vi "Clock Cross Retrieve.vi"(2 "resources":T2) -> (4 "read completion out":T1)   [LabVIEW 2020]
doc: "Retrieves the read completion from the other clock domain.\n\n<B>Input Parameters</B>\n\n<B>resources</B> contains references to the clock crossing FIFOs.\n\n<B>reset</B> is the register bus's reset signal.\n\n<B>Output Parameters</B>\n\n<B>read completion</B> the read completion data from the other clock domain.\n\n<B>ready for input</B> is a flow control signal that indicates whether the other clock domain's process is ready to accept a new instruction."
uses:
  Clock Cross Resources.ctl
  <instrlib>/_niInstr/Register Bus/v1/FPGA/Public/Read Completion.ctl
  <vilib>/rvi/DataTransferAndStorage/Container/Common/niFpgaContainerExecOnDevCompGetState.vi
  <vilib>/rvi/Emulation/niFpgaEmulationIsFPGAContextNoSignature.vi
  <vilib>/rvi/DataTransferAndStorage/Container/Common/niFpgaContainerGetUniqueNameForEmu.vi
  <vilib>/rvi/eio/common/nirviEmuReportErrorAndStop.vi
  <vilib>/rvi/Emulation/niFpgaSctlEmulationGetInTimedLoop.vi
  <vilib>/rvi/Emulation/niFpgaProcessEmulError.vi
  <vilib>/rvi/DataTransferAndStorage/Container/XNode/niFpgaContainer.xnode
  <vilib>/rvi/DataTransferAndStorage/Handshake/Emulation/niFpgaHandshakeEmulationRefIn.vi
  <instrlib>/_niInstr/Register Bus/v1/FPGA/niInstr Register Bus v1 FPGA.lvlib
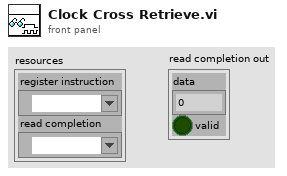
[diagram p1: front panel]
types:
  T1 = typedef "niInstr Register Bus v1 FPGA.lvlib/Read Completion.ctl" = cluster{"data":u32, "valid":bool}
  T2 = typedef "Clock Cross Resources.ctl" = cluster{"register instruction":refnum<k21>, "read completion":refnum<k21>}
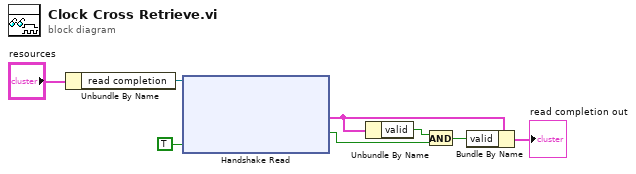
[diagram p0: block diagram]
diagram:
  n1 = Unbundle By Name("resources") -> ("read completion"=w4:refnum<k21>)
  n2 = xnode "Handshake Read"("Ready for Output"=TRUE ("ready for output"), "Handshake In"=w4) -> ("Data"=w1:cluster{"data":u32, "valid":bool}, "Output Valid"=w2:bool)  [unwired: 1 out]
  n3 = Unbundle By Name(w1) -> ("valid"=w7:bool)
  n4 = And(x=w7, y=w2) -> (x .and. y?=w6:bool)
  n5 = Bundle By Name(cluster=w1, "valid"=w6) -> (→"read completion out":cluster{"data":u32, "valid":bool})
